vi "master_stop.vi"() -> ()   [LabVIEW 2017]
panel:
  in  "MasterStop":bool
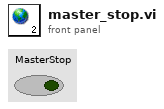
[diagram p1: front panel]
diagram:
